vi "Datacluster remove duplicates_sort.vi"(6 "tolerance":dbl=0.0005 format="%.3e", 7 "ascending":bool, 9 "Sort?":bool, 10 "Datasets to be processed":T3(array[cluster])=[{"String"="KR6_Rh3In3Ge4", "Boolean"=TRUE, "begin"=0, "length"=99, "y weight"=1.0}], 11 "data cluster":cluster{"all rows":dbl[][]}[](array[cluster])=[{"all rows"=[[292.0, 292.9164, 75.02219, 292.5198, 292.873, 0.08675399, 165.5123, 4.898979, 292.4821, 292.7706, 292.492, 292.5008, 293.2383, 292.873, 25.04327, 12.87815, 8.722502e-06, 147301.0, 0.0, 49.12202, 7.026817e-06], [292.0, 292.6799, 51.88008, 291.997, 292.6172, 0.1254523, 164.8345, 4.898979, 291.9992, 292.2308, 292.069, 291.9987, 292.9044, 292.6172, 16.68079, 8.502932, 7.87955e-06, 148972.5, 0.0, 52.73522, 7.82408e-06], [289.0, 289.5872, 53.36827, 288.998, 289.5262, 0.121954, 164.6135, 4.898979, 288.9966, 289.0375, 288.9818, 288.9977, 289.7039, 289.5262, 16.9019, 8.586199, 8.115929e-06, 149524.0, 0.0, 53.28857, 7.979706e-06], [286.0, 286.5259, 49.68945, 285.998, 286.4604, 0.130983, 164.4479, 4.898979, 285.9991, 285.8497, 285.9015, 285.9993, 286.5396, 286.4604, 16.3069, 8.351839, 7.550718e-06, 150070.2, 0.0, 49.26372, 7.019865e-06], [283.0, 283.4711, 53.72872, 283.0, 283.4105, 0.1211359, 164.3414, 4.898979, 282.9993, 282.7069, 282.8492, 283.0001, 283.3894, 283.4105, 16.49914, 8.324846, 8.321034e-06, 150632.6, 0.0, 53.01569, 7.9647e-06], [280.0, 280.4225, 55.74425, 280.001, 280.3641, 0.116756, 164.0834, 4.898979, 279.9989, 279.5874, 279.805, 279.9995, 280.2632, 280.3641, 16.65599, 8.355238, 8.692565e-06, 151182.8, 0.0, 57.0127, 8.356655e-06], [277.0, 277.4087, 53.59749, 277.0, 277.348, 0.1214324, 163.8697, 4.898979, 276.999, 276.4814, 276.7861, 277.0003, 277.1648, 277.348, 16.48811, 8.322479, 8.417088e-06, 151713.2, 0.0, 56.02918, 8.50766e-06], [274.0, 274.42, 54.6898, 274.001, 274.3605, 0.1190071, 163.7107, 4.898979, 273.9996, 273.4294, 273.7956, 274.0001, 274.1133, 274.3605, 16.45529, 8.266658, 8.774592e-06, 152257.0, 0.0, 55.53214, 8.58475e-06], [271.0, 271.4452, 55.7095, 271.001, 271.3868, 0.1168288, 163.585, 4.898979, 270.9994, 270.3922, 270.812, 270.9999, 271.0838, 271.3868, 16.27431, 8.125881, 8.904832e-06, 152814.4, 0.0, 56.2198, 8.635062e-06], [268.0, 268.4699, 56.23065, 268.001, 268.412, 0.115746, 163.4811, 4.898979, 267.9992, 267.3543, 267.8305, 267.9997, 268.0515, 268.412, 16.14259, 8.031859, 9.125312e-06, 153358.0, 0.0, 56.47631, 9.315139e-06], [265.0, 265.504, 56.7819, 265.0, 265.4467, 0.1146223, 163.391, 4.898979, 264.9995, 264.3426, 264.8619, 264.9997, 265.042, 265.4467, 16.08378, 7.981424, 9.334535e-06, 153898.2, 0.0, 56.33507, 9.071532e-06], [262.0, 262.5402, 56.3029, 261.999, 262.4824, 0.1155975, 163.3034, 4.898979, 261.9999, 261.3382, 261.8933, 262.0, 262.0429, 262.4824, 15.96119, 7.921869, 9.410211e-06, 154447.6, 0.0, 56.37045, 9.069828e-06], [259.0, 259.5962, 58.10709, 259.0, 259.5401, 0.1120083, 163.2193, 4.898979, 258.9994, 258.3609, 258.9463, 258.9997, 259.0668, 259.5401, 15.93857, 7.860623, 9.705625e-06, 154984.0, 0.0, 56.57644, 9.146704e-06], [256.0, 256.6687, 56.23365, 255.999, 256.6109, 0.1157399, 163.1493, 4.898979, 255.999, 255.398, 256.0085, 255.9989, 256.1162, 256.6109, 15.6581, 7.744409, 9.492895e-06, 155529.5, 0.0, 56.48109, 9.279682e-06], [253.0, 253.5733, 56.38813, 253.0, 253.53, 0.08656709, 163.0587, 4.242641, 252.9989, 252.4462, 253.0724, 252.9998, 252.9904, 253.53, 15.52846, 7.664103, 9.532705e-06, 156076.4, 0.0, 55.89689, 9.252784e-06], [250.0, 250.6412, 54.69462, 250.0, 250.5966, 0.08924747, 162.9786, 4.242641, 250.0002, 249.4823, 250.1305, 250.0004, 250.0376, 250.5966, 15.19496, 7.512066, 9.061377e-06, 156639.2, 0.0, 56.67262, 9.431853e-06], [247.0, 247.7008, 56.19418, 247.001, 247.6573, 0.08686587, 162.8957, 4.242641, 246.9987, 246.5324, 247.1849, 247.0003, 247.0917, 247.6573, 15.12285, 7.431846, 9.658179e-06, 157187.5, 0.0, 58.88652, 9.951588e-06], [244.0, 244.756, 57.27194, 243.999, 244.7134, 0.08523119, 162.8167, 4.242641, 243.9985, 243.5809, 244.2381, 243.9991, 244.1415, 244.7134, 15.06449, 7.372421, 1.015879e-05, 157736.6, 0.0, 57.34745, 9.89733e-06], [241.0, 241.8457, 56.35606, 240.999, 241.8024, 0.08661635, 162.7319, 4.242641, 240.9999, 240.6596, 241.3181, 240.9994, 241.2305, 241.8024, 14.76138, 7.218644, 1.001309e-05, 158281.2, 0.0, 55.59713, 9.467991e-06], [238.0, 238.9209, 56.78944, 238.0, 238.8779, 0.08595534, 162.6528, 4.242641, 237.9983, 237.7335, 238.3869, 237.9997, 238.3104, 238.8779, 14.65413, 7.147241, 9.925203e-06, 158821.8, 0.0, 57.4055, 9.991189e-06], [235.0, 235.8546, 58.50336, 235.0, 235.8233, 0.0625779, 162.5361, 3.674235, 234.9997, 234.8069, 235.452, 234.9992, 235.2407, 235.8233, 14.56547, 7.060409, 1.032292e-05, 159362.6, 0.0, 58.88609, 1.077016e-05], [232.0, 232.9135, 58.7887, 232.0, 232.8823, 0.06227416, 162.4497, 3.674235, 231.9992, 231.8697, 232.505, 232.0, 232.3093, 232.8823, 14.4148, 6.969601, 1.039831e-05, 159894.4, 0.0, 60.38943, 1.099243e-05], [229.0, 229.9683, 52.90027, 228.999, 229.9337, 0.06920602, 162.3651, 3.674235, 228.9996, 228.9262, 229.5497, 228.9995, 229.3795, 229.9337, 13.95679, 6.834046, 9.47672e-06, 160443.8, 0.0, 55.18934, 1.011709e-05], [226.0, 227.0314, 55.01033, 226.001, 226.9982, 0.06655145, 162.2802, 3.674235, 225.9986, 225.9999, 226.6072, 226.0003, 226.4574, 226.9982, 13.87658, 6.741458, 1.003314e-05, 160986.4, 0.0, 56.71966, 9.916942e-06], [223.0, 224.0942, 54.51703, 222.999, 224.0606, 0.06715364, 162.193, 3.674235, 222.9989, 223.0755, 223.6635, 222.999, 223.5397, 224.0606, 13.63051, 6.611919, 9.828761e-06, 161551.5, 0.0, 57.5095, 1.147469e-05], [220.0, 221.1488, 53.22712, 219.999, 221.1144, 0.06878105, 162.1079, 3.674235, 219.9987, 220.1357, 220.7061, 219.9996, 220.6128, 221.1144, 13.28219, 6.44084, 9.954398e-06, 162102.9, 0.0, 56.94044, 1.050179e-05], [217.0, 218.18, 55.6197, 217.0, 218.1471, 0.06582231, 162.0181, 3.674235, 216.9999, 217.1911, 217.7388, 216.9998, 217.6652, 218.1471, 13.33998, 6.426719, 1.030691e-05, 162650.0, 0.0, 54.95497, 1.056938e-05], [214.0, 215.2041, 52.74785, 214.001, 215.1694, 0.069406, 161.9245, 3.674235, 213.9993, 214.2305, 214.7574, 214.0001, 214.7119, 215.1694, 13.16094, 6.381908, 1.041787e-05, 163183.7, 0.0, 54.82949, 1.00501e-05], [211.0, 212.2438, 53.2594, 210.999, 212.2094, 0.06873936, 161.8459, 3.674235, 211.0002, 211.2871, 211.7895, 210.9995, 211.7758, 212.2094, 12.92852, 6.240668, 1.038931e-05, 163737.5, 0.0, 53.69054, 9.725446e-06], [208.0, 209.2728, 54.18705, 208.0, 209.239, 0.06756258, 161.7569, 3.674235, 207.9997, 208.341, 208.8189, 207.9994, 208.8287, 209.239, 12.96622, 6.244319, 1.030433e-05, 164296.5, 0.0, 51.99244, 9.937355e-06], [205.0, 206.3015, 47.85468, 204.999, 206.2633, 0.0765028, 161.669, 3.674235, 204.9996, 205.3777, 205.8335, 204.9997, 205.8839, 206.2633, 12.49721, 6.108157, 8.850608e-06, 164832.5, 0.0, 52.33099, 1.025279e-05], [202.0, 203.3115, 47.77909, 202.0, 203.2732, 0.07662382, 161.578, 3.674235, 201.9992, 202.4024, 202.836, 201.9998, 202.9163, 203.2732, 12.32563, 6.011273, 9.175306e-06, 165383.8, 0.0, 49.48042, 9.796374e-06], [199.0, 200.3016, 48.81196, 199.001, 200.2641, 0.07500245, 161.4837, 3.674235, 198.9994, 199.4091, 199.8188, 199.0009, 199.9294, 200.2641, 12.19196, 5.913105, 9.19541e-06, 165931.2, 0.0, 48.99235, 9.119814e-06], [196.0, 197.3124, 46.33101, 196.0, 197.2728, 0.07901871, 161.3904, 3.674235, 195.9999, 196.4343, 196.8208, 195.9996, 196.9654, 197.2728, 11.90443, 5.801792, 9.14851e-06, 166481.8, 0.0, 47.56836, 9.084771e-06], [193.0, 194.3294, 48.48906, 193.0, 194.2917, 0.07550192, 161.2938, 3.674235, 192.9996, 193.4505, 193.8166, 192.9997, 194.001, 194.2917, 11.49295, 5.526408, 9.320439e-06, 167039.8, 0.0, 49.01581, 9.34799e-06], [190.0, 191.3157, 47.75745, 189.999, 191.2773, 0.07665855, 161.2094, 3.674235, 190.0005, 190.4523, 190.7964, 189.9991, 191.0099, 191.2773, 11.31843, 5.442408, 9.51165e-06, 167586.2, 0.0, 47.72681, 9.290438e-06], [187.0, 188.2909, 46.66995, 186.998, 188.2517, 0.07844485, 161.1183, 3.674235, 186.9996, 187.4401, 187.7654, 187.0006, 188.0048, 188.2517, 11.22194, 5.408542, 9.210011e-06, 168125.0, 0.0, 47.7442, 9.335471e-06], [184.0, 185.2608, 45.59003, 184.0, 185.2207, 0.08030301, 161.02, 3.674235, 183.9996, 184.4185, 184.7246, 183.9997, 184.9949, 185.2207, 10.97692, 5.291597, 8.987941e-06, 168671.0, 0.0, 45.18603, 8.882518e-06], [181.0, 182.2488, 42.55964, 181.0, 182.2057, 0.08602087, 160.9233, 3.674235, 180.9996, 181.4114, 181.7032, 180.9994, 182.0001, 182.2057, 10.7433, 5.21988, 8.481294e-06, 169224.8, 0.0, 42.92117, 8.932989e-06], [178.0, 179.2327, 43.4817, 178.0, 179.1906, 0.08419672, 160.8244, 3.674235, 177.9992, 178.3866, 178.6756, 177.9989, 178.9857, 179.1906, 10.55317, 5.093926, 8.674955e-06, 169761.4, 0.0, 46.08075, 9.801831e-06], [175.0, 176.1988, 41.91763, 174.999, 176.1551, 0.08733836, 160.7272, 3.674235, 174.9992, 175.3492, 175.6323, 175.0005, 175.9594, 176.1551, 10.39018, 5.032765, 8.418331e-06, 170337.0, 0.0, 41.27729, 8.256854e-06], [172.0, 173.1462, 40.78401, 171.998, 173.1014, 0.08976599, 160.6309, 3.674235, 171.9994, 172.2934, 172.5681, 172.0007, 172.9165, 173.1014, 10.17369, 4.933174, 8.561175e-06, 170884.7, 0.0, 42.0311, 8.954053e-06], [169.0, 170.1156, 39.52542, 169.002, 170.0692, 0.09262438, 160.5319, 3.674235, 168.9985, 169.2597, 169.5281, 169.0004, 169.8935, 170.0692, 10.01111, 4.866947, 7.889127e-06, 171427.6, 0.0, 41.17875, 8.476864e-06], [166.0, 167.0848, 37.75683, 166.0, 167.0363, 0.09696304, 160.4351, 3.674235, 165.9992, 166.2177, 166.4835, 165.9991, 166.8676, 167.0363, 9.732579, 4.745978, 7.667965e-06, 171976.2, 0.0, 40.17138, 7.923543e-06], [163.0, 164.0348, 37.48756, 163.0, 163.986, 0.09765951, 160.3364, 3.674235, 162.9994, 163.1585, 163.4224, 162.9994, 163.8198, 163.986, 9.565177, 4.656068, 7.403833e-06, 172519.0, 0.0, 37.92251, 7.706918e-06], [160.0, 160.9789, 37.24322, 160.0, 160.9297, 0.09830023, 160.2345, 3.674235, 159.9997, 160.0851, 160.3523, 159.9997, 160.7607, 160.9297, 9.362346, 4.545693, 7.846706e-06, 173077.8, 0.0, 38.13007, 8.027448e-06], [157.0, 157.7978, 36.56221, 157.0, 157.7603, 0.07509838, 160.1422, 3.181981, 157.0001, 157.0355, 157.3161, 157.0001, 157.5547, 157.7603, 9.136679, 4.431653, 7.299468e-06, 173622.6, 0.0, 36.74182, 7.431135e-06], [154.0, 154.7562, 36.11287, 153.999, 154.7182, 0.0760328, 160.039, 3.181981, 154.0002, 153.9788, 154.2641, 153.9991, 154.5089, 154.7182, 8.931389, 4.324545, 7.829839e-06, 174165.6, 0.0, 37.11626, 7.907207e-06], [151.0, 151.7025, 35.56308, 151.001, 151.6639, 0.07720823, 159.94, 3.181981, 150.9997, 150.9063, 151.1997, 151.0003, 151.4478, 151.6639, 8.772177, 4.245581, 7.074522e-06, 174712.4, 0.0, 34.8322, 7.606191e-06], [148.0, 148.6425, 34.07633, 148.001, 148.6022, 0.08057683, 159.8368, 3.181981, 148.0007, 147.8203, 148.1272, 148.0007, 148.376, 148.6022, 8.538666, 4.143502, 7.012669e-06, 175270.5, 0.0, 35.5259, 7.773223e-06], [145.0, 145.6151, 32.94494, 145.0, 145.5734, 0.08334398, 159.7329, 3.181981, 144.9995, 144.7711, 145.0917, 145.0, 145.3362, 145.5734, 8.402115, 4.089585, 6.717016e-06, 175825.6, 0.0, 34.5873, 7.462285e-06], [142.0, 142.4503, 32.69128, 141.998, 142.4188, 0.062993, 159.6235, 2.755676, 141.9999, 141.7087, 142.045, 141.998, 142.1454, 142.4188, 8.112161, 3.93007, 6.970786e-06, 176365.9, 0.0, 33.20516, 7.879391e-06], [139.0, 139.3994, 31.76623, 139.001, 139.367, 0.06482741, 159.5169, 2.755676, 138.9981, 138.6308, 138.9849, 138.9994, 139.0777, 139.367, 7.985541, 3.877216, 6.982463e-06, 176903.8, 0.0, 32.45839, 6.596733e-06], [136.0, 136.3652, 31.01851, 135.998, 136.332, 0.0663901, 159.4101, 2.755676, 135.9989, 135.5674, 135.9417, 135.999, 136.0241, 136.332, 7.79429, 3.784086, 6.795836e-06, 177452.3, 0.0, 32.19581, 6.462182e-06], [133.0, 133.3502, 30.5601, 133.0, 133.3165, 0.06738596, 159.3015, 2.755676, 132.9992, 132.5206, 132.9147, 132.9999, 132.9898, 133.3165, 7.59515, 3.680558, 6.903421e-06, 178000.4, 0.0, 31.58324, 6.744551e-06], [130.0, 130.2115, 29.16558, 130.0, 130.185, 0.05295598, 159.122, 2.386485, 130.0005, 129.4585, 129.875, 129.9997, 129.8214, 130.185, 7.33831, 3.563506, 7.084772e-06, 178528.9, 0.0, 30.31422, 6.637657e-06], [127.0, 127.0902, 28.66261, 127.0, 127.07, 0.04041393, 159.0379, 2.066757, 126.9998, 126.3926, 126.8334, 126.9993, 126.6696, 127.07, 7.211448, 3.501876, 6.550803e-06, 179072.6, 0.0, 27.84635, 6.955272e-06], [124.0, 124.092, 28.58992, 124.0, 124.0717, 0.04051669, 158.9287, 2.066757, 124.0006, 123.3645, 123.8279, 123.9994, 123.6488, 124.0717, 7.012868, 3.390962, 7.173261e-06, 179624.9, 0.0, 28.22442, 4.92486e-06], [121.0, 121.0173, 26.81918, 120.999, 121.0011, 0.03239384, 158.8124, 1.789864, 120.9991, 120.3247, 120.8123, 120.9995, 120.5459, 121.0011, 6.797255, 3.304885, 4.45575e-06, 180140.8, 0.0, 29.19013, 5.915953e-06], [118.0, 117.9932, 25.80576, 117.999, 117.9764, 0.03366599, 158.6989, 1.789864, 117.9995, 117.2703, 117.781, 118.0, 117.4994, 117.9764, 6.568201, 3.195852, 5.482144e-06, 180683.1, 0.0, 27.08986, 6.913137e-06], [115.0, 115.0141, 25.65538, 114.998, 114.9971, 0.03386332, 158.5865, 1.789864, 115.0005, 114.2643, 114.7982, 114.9996, 114.497, 114.9971, 6.423356, 3.116589, 5.528924e-06, 181217.8, 0.0, 26.62919, 5.253105e-06], [112.0, 112.0203, 26.59349, 112.001, 112.004, 0.03266877, 158.4708, 1.789864, 111.9995, 111.2424, 111.7992, 111.9994, 111.4798, 112.004, 6.320665, 3.040642, 5.840544e-06, 181744.4, 0.0, 26.32533, 6.485414e-06], [109.0, 109.016, 25.89338, 109.0, 108.9992, 0.03355207, 158.3582, 1.789864, 109.0002, 108.2095, 108.7884, 108.9998, 108.4539, 108.9992, 6.13315, 2.948822, 4.976681e-06, 182293.6, 0.0, 25.56833, 6.586255e-06], [106.0, 106.0601, 24.74948, 105.999, 106.0426, 0.03510282, 158.2417, 1.789864, 106.0009, 105.2233, 105.8221, 105.9986, 105.4789, 106.0426, 5.82098, 2.795607, 5.520496e-06, 182820.9, 0.0, 25.1926, 5.082759e-06], [103.0, 103.1012, 23.47957, 102.999, 103.0827, 0.03700138, 158.1265, 1.789864, 102.9994, 102.2249, 102.852, 102.9995, 102.4926, 103.0827, 5.610787, 2.701479, 5.748678e-06, 183358.4, 0.0, 24.56658, 4.990891e-06], [100.0, 100.1194, 24.40213, 100.0, 100.1016, 0.03560248, 158.0093, 1.789864, 99.99963, 99.21942, 99.86005, 99.99973, 99.49659, 100.1016, 5.418124, 2.579388, 5.193695e-06, 183898.6, 0.0, 24.73305, 4.828259e-06], [97.0, 97.17382, 23.39176, 97.0015, 97.15525, 0.03714027, 157.8955, 1.789864, 96.99884, 96.25454, 96.90598, 96.99946, 96.54095, 97.15525, 5.252876, 2.504921, 5.62191e-06, 184439.7, 0.0, 23.73066, 5.229691e-06], [94.0, 94.20774, 23.22087, 94.0002, 94.18903, 0.0374136, 157.7782, 1.789864, 93.99808, 93.27039, 93.92858, 94.00004, 93.56826, 94.18903, 5.073145, 2.409457, 5.538685e-06, 184984.4, 0.0, 23.61211, 6.687232e-06], [91.0, 91.13359, 22.59694, 91.0003, 91.11917, 0.02883498, 157.6522, 1.550068, 91.0004, 90.31659, 90.91559, 90.9996, 90.54901, 91.11917, 4.827745, 2.285596, 4.255465e-06, 185533.6, 0.0, 21.92768, 5.296259e-06], [88.0, 88.18123, 22.48137, 87.9991, 88.16674, 0.02898322, 157.5325, 1.550068, 87.9996, 87.35154, 87.95371, 87.99927, 87.59355, 88.16674, 4.645815, 2.189353, 4.903361e-06, 186084.2, 0.0, 21.34062, 6.20428e-06], [85.0, 85.24232, 22.00163, 84.9979, 85.22751, 0.02961518, 157.4127, 1.550068, 85.00029, 84.40605, 85.0051, 84.99872, 84.65807, 85.22751, 4.439868, 2.085645, 3.898806e-06, 186641.8, 0.0, 20.03455, 4.048067e-06], [82.0, 82.2906, 20.26436, 82.0003, 82.27452, 0.0321541, 157.2935, 1.550068, 81.99943, 81.3944, 82.04882, 81.99944, 81.65225, 82.27452, 4.366601, 2.069786, 4.384861e-06, 187170.4, 0.0, 19.93068, 5.169709e-06], [79.0, 79.35992, 20.65986, 78.9998, 79.34415, 0.03153857, 157.175, 1.550068, 78.99976, 78.46501, 79.10271, 78.99972, 78.73799, 79.34415, 4.123809, 1.934396, 5.660535e-06, 187707.0, 0.0, 20.24228, 3.521332e-06], [76.0, 76.34799, 18.14755, 76.0001, 76.33453, 0.02692852, 157.0442, 1.342398, 75.9988, 75.52364, 76.14176, 76.00082, 75.74333, 76.33453, 3.879228, 1.836679, 5.277406e-06, 188227.8, 0.0, 18.3202, 4.280038e-06], [73.0, 73.40674, 18.83722, 72.9989, 73.39377, 0.02594261, 156.9286, 1.342398, 72.9991, 72.60294, 73.19315, 72.99918, 72.82951, 73.39377, 3.728216, 1.746902, 4.133453e-06, 188764.6, 0.0, 20.32012, 4.874801e-06], [70.0, 70.45695, 17.51673, 70.0003, 70.443, 0.02789829, 156.8115, 1.342398, 70.00086, 69.67221, 70.23128, 69.99956, 69.91183, 70.443, 3.505012, 1.644658, 3.415282e-06, 189312.8, 0.0, 18.10538, 3.636672e-06], [67.0, 67.51137, 17.06142, 66.9986, 67.49705, 0.0286428, 156.6926, 1.342398, 67.0003, 66.75251, 67.27265, 66.99976, 67.00556, 67.49705, 3.329935, 1.557489, 3.637388e-06, 189850.0, 0.0, 17.81273, 2.997229e-06], [64.0, 64.55299, 16.05667, 63.9994, 64.53777, 0.03043512, 156.572, 1.342398, 63.99965, 63.82388, 64.3001, 64.00019, 64.09199, 64.53777, 3.155975, 1.477454, 3.836114e-06, 190372.4, 0.0, 16.65761, 3.137167e-06], [61.0, 61.59684, 15.15327, 61.0012, 61.58071, 0.03224959, 156.4552, 1.342398, 61.00003, 60.89696, 61.32582, 60.99921, 61.18411, 61.58071, 2.932403, 1.370073, 2.715446e-06, 190890.4, 0.0, 15.46223, 4.794554e-06], [58.0, 58.6279, 14.0184, 58.0008, 58.61047, 0.03486038, 156.3434, 1.342398, 57.99915, 57.96364, 58.33762, 57.99934, 58.27135, 58.61047, 2.745862, 1.284894, 2.94282e-06, 191408.4, 0.0, 14.4151, 4.772166e-06], [55.0, 55.65962, 12.33515, 55.0029, 55.63981, 0.03961743, 156.2312, 1.342398, 54.99762, 55.02696, 55.34105, 55.0008, 55.36534, 55.63981, 2.519189, 1.185287, 3.164869e-06, 191919.5, 0.0, 12.86659, 1.828514e-06], [52.0, 52.69421, 11.21244, 51.999, 52.67242, 0.04358434, 156.12, 1.342398, 51.99888, 52.0955, 52.34609, 51.99949, 52.46542, 52.67242, 2.286444, 1.075562, 2.081657e-06, 192439.7, 0.0, 11.76603, 2.789106e-06], [49.0, 49.61418, 9.645293, 49.001, 49.59518, 0.03799937, 156.0042, 1.162551, 48.99919, 49.13845, 49.32293, 49.00038, 49.4487, 49.59518, 2.049105, 0.9693383, 2.419945e-06, 192925.6, 0.0, 10.21014, 2.551699e-06], [46.0, 46.64398, 8.849838, 46.0014, 46.62327, 0.04141489, 155.8991, 1.162551, 45.99971, 46.20159, 46.31906, 45.99925, 46.54721, 46.62327, 1.829977, 0.8624549, 2.062263e-06, 193484.8, 0.0, 8.642792, 8.766135e-07], [43.0, 43.63805, 8.111564, 43.0, 43.61546, 0.04518427, 155.7963, 1.162551, 43.00087, 43.23263, 43.28277, 42.99939, 43.6105, 43.61546, 1.669476, 0.7863123, 2.202847e-06, 194031.9, 0.0, 8.304894, 2.187056e-06], [40.0, 40.60721, 7.850611, 39.9976, 40.58387, 0.04668618, 155.6928, 1.162551, 39.99903, 40.24392, 40.22946, 39.99922, 40.64502, 40.58387, 1.579687, 0.7417823, 1.934699e-06, 194511.3, 0.0, 7.823251, 1.052641e-06], [37.0, 37.55588, 7.570818, 37.0021, 37.53168, 0.04841156, 155.5887, 1.162551, 36.99997, 37.23081, 37.15568, 36.99985, 37.65521, 37.53168, 1.491856, 0.6986331, 1.616464e-06, 195029.6, 0.0, 7.701154, 1.426829e-06], [34.0, 34.39013, 7.129456, 34.002, 34.37085, 0.03855642, 155.4653, 1.006799, 34.00288, 34.19961, 34.07078, 33.99971, 34.53824, 34.37085, 1.389701, 0.6498903, 1.456064e-06, 195501.9, 0.0, 7.197325, 1.830936e-06], [31.0, 31.3295, 6.959681, 30.9971, 31.30975, 0.03949697, 155.3693, 1.006799, 31.00027, 31.15947, 30.98673, 30.99905, 31.52198, 31.30975, 1.305866, 0.6077944, 1.746532e-06, 195974.6, 0.0, 6.855044, 1.3535e-07], [28.0, 28.257, 6.444445, 28.0083, 28.23568, 0.04265477, 155.2754, 1.006799, 27.99751, 28.08427, 27.88122, 28.00025, 28.48138, 28.23568, 1.20443, 0.5603139, 1.207888e-06, 196438.7, 0.0, 6.465166, 2.29124e-06], [25.0, 25.1858, 5.908139, 25.0055, 25.16253, 0.04652672, 155.1906, 1.006799, 25.00147, 24.99086, 24.77406, 24.99832, 25.42586, 25.16253, 1.084087, 0.5032175, 9.614257e-07, 196931.6, 0.0, 5.92471, -5.51895e-08], [22.0, 22.16916, 5.305623, 21.9854, 22.14325, 0.05181037, 155.1142, 1.006799, 22.00671, 21.91764, 21.70696, 21.99982, 22.40575, 22.14325, 0.959603, 0.4446781, 7.916026e-07, 197380.4, 0.0, 5.277611, 2.768679e-07], [19.0, 19.30572, 4.637635, 18.9844, 19.27608, 0.05927295, 155.0499, 1.006799, 18.99661, 18.95241, 18.76765, 19.00061, 19.52011, 19.27608, 0.8426237, 0.390679, 5.587576e-07, 197860.4, 0.0, 4.670142, -7.621961e-08], [16.0, 16.50024, 3.972702, 16.0034, 16.46565, 0.06919378, 154.9962, 1.006799, 15.99681, 16.00464, 15.86607, 15.99389, 16.67341, 16.46565, 0.7071578, 0.3270905, 3.955843e-07, 198345.2, 0.0, 3.981336, -9.093087e-09], [13.0, 13.71888, 3.255681, 13.0265, 13.67666, 0.08443282, 154.9529, 1.006799, 12.99021, 12.98951, 12.9155, 12.99523, 13.83511, 13.67666, 0.5650661, 0.2606204, 4.899574e-08, 199058.5, 0.0, 3.267024, -3.089664e-07], [10.0, 11.02144, 2.634719, 9.9178, 10.96927, 0.1043323, 154.9244, 1.006799, 9.979209, 9.944225, 9.937939, 9.981572, 11.07989, 10.96927, 0.4191188, 0.1915213, 3.509129e-08, 199788.6, 0.0, 2.637912, 3.892924e-07], [7.0, 8.207977, 2.280254, 7.0263, 8.162771, 0.09041306, 154.877, 0.8719131, 6.996675, 6.899136, 6.944581, 6.995916, 8.207738, 8.162771, 0.272072, 0.1212537, 1.590448e-07, 200474.8, 0.0, 2.226699, -2.06841e-07], [4.0, 6.17061, 6.914511, 3.9852, 6.155702, 0.02981624, 154.8519, 0.8719131, 4.007358, 3.946248, 3.912001, 4.007225, 6.219766, 6.155702, 0.1566822, 0.06587024, 3.496313e-07, 201190.7, 0.0, 6.388795, -3.268214e-08], [2.0, 3.439481, -0.8426919, 2.2818, 3.470062, -0.06116255, 154.8119, 0.4359565, 2.275721, 2.314741, 2.136495, 2.275818, 3.587147, 3.470062, 0.06999886, 0.02771, -3.623877e-09, 201712.2, 0.0, -0.8426919, -3.623877e-09]]}]) -> (3 "data cluster out":cluster{"all rows":dbl[][]}[](array[cluster])=[{"all rows"=[[292.0, 292.9164, 75.02219, 292.5198, 292.873, 0.08675399, 165.5123, 4.898979, 292.4821, 292.7706, 292.492, 292.5008, 293.2383, 292.873, 25.04327, 12.87815, 8.722502e-06, 147301.0, 0.0, 49.12202, 7.026817e-06], [292.0, 292.6799, 51.88008, 291.997, 292.6172, 0.1254523, 164.8345, 4.898979, 291.9992, 292.2308, 292.069, 291.9987, 292.9044, 292.6172, 16.68079, 8.502932, 7.87955e-06, 148972.5, 0.0, 52.73522, 7.82408e-06], [289.0, 289.5872, 53.36827, 288.998, 289.5262, 0.121954, 164.6135, 4.898979, 288.9966, 289.0375, 288.9818, 288.9977, 289.7039, 289.5262, 16.9019, 8.586199, 8.115929e-06, 149524.0, 0.0, 53.28857, 7.979706e-06], [286.0, 286.5259, 49.68945, 285.998, 286.4604, 0.130983, 164.4479, 4.898979, 285.9991, 285.8497, 285.9015, 285.9993, 286.5396, 286.4604, 16.3069, 8.351839, 7.550718e-06, 150070.2, 0.0, 49.26372, 7.019865e-06], [283.0, 283.4711, 53.72872, 283.0, 283.4105, 0.1211359, 164.3414, 4.898979, 282.9993, 282.7069, 282.8492, 283.0001, 283.3894, 283.4105, 16.49914, 8.324846, 8.321034e-06, 150632.6, 0.0, 53.01569, 7.9647e-06], [280.0, 280.4225, 55.74425, 280.001, 280.3641, 0.116756, 164.0834, 4.898979, 279.9989, 279.5874, 279.805, 279.9995, 280.2632, 280.3641, 16.65599, 8.355238, 8.692565e-06, 151182.8, 0.0, 57.0127, 8.356655e-06], [277.0, 277.4087, 53.59749, 277.0, 277.348, 0.1214324, 163.8697, 4.898979, 276.999, 276.4814, 276.7861, 277.0003, 277.1648, 277.348, 16.48811, 8.322479, 8.417088e-06, 151713.2, 0.0, 56.02918, 8.50766e-06], [274.0, 274.42, 54.6898, 274.001, 274.3605, 0.1190071, 163.7107, 4.898979, 273.9996, 273.4294, 273.7956, 274.0001, 274.1133, 274.3605, 16.45529, 8.266658, 8.774592e-06, 152257.0, 0.0, 55.53214, 8.58475e-06], [271.0, 271.4452, 55.7095, 271.001, 271.3868, 0.1168288, 163.585, 4.898979, 270.9994, 270.3922, 270.812, 270.9999, 271.0838, 271.3868, 16.27431, 8.125881, 8.904832e-06, 152814.4, 0.0, 56.2198, 8.635062e-06], [268.0, 268.4699, 56.23065, 268.001, 268.412, 0.115746, 163.4811, 4.898979, 267.9992, 267.3543, 267.8305, 267.9997, 268.0515, 268.412, 16.14259, 8.031859, 9.125312e-06, 153358.0, 0.0, 56.47631, 9.315139e-06], [265.0, 265.504, 56.7819, 265.0, 265.4467, 0.1146223, 163.391, 4.898979, 264.9995, 264.3426, 264.8619, 264.9997, 265.042, 265.4467, 16.08378, 7.981424, 9.334535e-06, 153898.2, 0.0, 56.33507, 9.071532e-06], [262.0, 262.5402, 56.3029, 261.999, 262.4824, 0.1155975, 163.3034, 4.898979, 261.9999, 261.3382, 261.8933, 262.0, 262.0429, 262.4824, 15.96119, 7.921869, 9.410211e-06, 154447.6, 0.0, 56.37045, 9.069828e-06], [259.0, 259.5962, 58.10709, 259.0, 259.5401, 0.1120083, 163.2193, 4.898979, 258.9994, 258.3609, 258.9463, 258.9997, 259.0668, 259.5401, 15.93857, 7.860623, 9.705625e-06, 154984.0, 0.0, 56.57644, 9.146704e-06], [256.0, 256.6687, 56.23365, 255.999, 256.6109, 0.1157399, 163.1493, 4.898979, 255.999, 255.398, 256.0085, 255.9989, 256.1162, 256.6109, 15.6581, 7.744409, 9.492895e-06, 155529.5, 0.0, 56.48109, 9.279682e-06], [253.0, 253.5733, 56.38813, 253.0, 253.53, 0.08656709, 163.0587, 4.242641, 252.9989, 252.4462, 253.0724, 252.9998, 252.9904, 253.53, 15.52846, 7.664103, 9.532705e-06, 156076.4, 0.0, 55.89689, 9.252784e-06], [250.0, 250.6412, 54.69462, 250.0, 250.5966, 0.08924747, 162.9786, 4.242641, 250.0002, 249.4823, 250.1305, 250.0004, 250.0376, 250.5966, 15.19496, 7.512066, 9.061377e-06, 156639.2, 0.0, 56.67262, 9.431853e-06], [247.0, 247.7008, 56.19418, 247.001, 247.6573, 0.08686587, 162.8957, 4.242641, 246.9987, 246.5324, 247.1849, 247.0003, 247.0917, 247.6573, 15.12285, 7.431846, 9.658179e-06, 157187.5, 0.0, 58.88652, 9.951588e-06], [244.0, 244.756, 57.27194, 243.999, 244.7134, 0.08523119, 162.8167, 4.242641, 243.9985, 243.5809, 244.2381, 243.9991, 244.1415, 244.7134, 15.06449, 7.372421, 1.015879e-05, 157736.6, 0.0, 57.34745, 9.89733e-06], [241.0, 241.8457, 56.35606, 240.999, 241.8024, 0.08661635, 162.7319, 4.242641, 240.9999, 240.6596, 241.3181, 240.9994, 241.2305, 241.8024, 14.76138, 7.218644, 1.001309e-05, 158281.2, 0.0, 55.59713, 9.467991e-06], [238.0, 238.9209, 56.78944, 238.0, 238.8779, 0.08595534, 162.6528, 4.242641, 237.9983, 237.7335, 238.3869, 237.9997, 238.3104, 238.8779, 14.65413, 7.147241, 9.925203e-06, 158821.8, 0.0, 57.4055, 9.991189e-06], [235.0, 235.8546, 58.50336, 235.0, 235.8233, 0.0625779, 162.5361, 3.674235, 234.9997, 234.8069, 235.452, 234.9992, 235.2407, 235.8233, 14.56547, 7.060409, 1.032292e-05, 159362.6, 0.0, 58.88609, 1.077016e-05], [232.0, 232.9135, 58.7887, 232.0, 232.8823, 0.06227416, 162.4497, 3.674235, 231.9992, 231.8697, 232.505, 232.0, 232.3093, 232.8823, 14.4148, 6.969601, 1.039831e-05, 159894.4, 0.0, 60.38943, 1.099243e-05], [229.0, 229.9683, 52.90027, 228.999, 229.9337, 0.06920602, 162.3651, 3.674235, 228.9996, 228.9262, 229.5497, 228.9995, 229.3795, 229.9337, 13.95679, 6.834046, 9.47672e-06, 160443.8, 0.0, 55.18934, 1.011709e-05], [226.0, 227.0314, 55.01033, 226.001, 226.9982, 0.06655145, 162.2802, 3.674235, 225.9986, 225.9999, 226.6072, 226.0003, 226.4574, 226.9982, 13.87658, 6.741458, 1.003314e-05, 160986.4, 0.0, 56.71966, 9.916942e-06], [223.0, 224.0942, 54.51703, 222.999, 224.0606, 0.06715364, 162.193, 3.674235, 222.9989, 223.0755, 223.6635, 222.999, 223.5397, 224.0606, 13.63051, 6.611919, 9.828761e-06, 161551.5, 0.0, 57.5095, 1.147469e-05], [220.0, 221.1488, 53.22712, 219.999, 221.1144, 0.06878105, 162.1079, 3.674235, 219.9987, 220.1357, 220.7061, 219.9996, 220.6128, 221.1144, 13.28219, 6.44084, 9.954398e-06, 162102.9, 0.0, 56.94044, 1.050179e-05], [217.0, 218.18, 55.6197, 217.0, 218.1471, 0.06582231, 162.0181, 3.674235, 216.9999, 217.1911, 217.7388, 216.9998, 217.6652, 218.1471, 13.33998, 6.426719, 1.030691e-05, 162650.0, 0.0, 54.95497, 1.056938e-05], [214.0, 215.2041, 52.74785, 214.001, 215.1694, 0.069406, 161.9245, 3.674235, 213.9993, 214.2305, 214.7574, 214.0001, 214.7119, 215.1694, 13.16094, 6.381908, 1.041787e-05, 163183.7, 0.0, 54.82949, 1.00501e-05], [211.0, 212.2438, 53.2594, 210.999, 212.2094, 0.06873936, 161.8459, 3.674235, 211.0002, 211.2871, 211.7895, 210.9995, 211.7758, 212.2094, 12.92852, 6.240668, 1.038931e-05, 163737.5, 0.0, 53.69054, 9.725446e-06], [208.0, 209.2728, 54.18705, 208.0, 209.239, 0.06756258, 161.7569, 3.674235, 207.9997, 208.341, 208.8189, 207.9994, 208.8287, 209.239, 12.96622, 6.244319, 1.030433e-05, 164296.5, 0.0, 51.99244, 9.937355e-06], [205.0, 206.3015, 47.85468, 204.999, 206.2633, 0.0765028, 161.669, 3.674235, 204.9996, 205.3777, 205.8335, 204.9997, 205.8839, 206.2633, 12.49721, 6.108157, 8.850608e-06, 164832.5, 0.0, 52.33099, 1.025279e-05], [202.0, 203.3115, 47.77909, 202.0, 203.2732, 0.07662382, 161.578, 3.674235, 201.9992, 202.4024, 202.836, 201.9998, 202.9163, 203.2732, 12.32563, 6.011273, 9.175306e-06, 165383.8, 0.0, 49.48042, 9.796374e-06], [199.0, 200.3016, 48.81196, 199.001, 200.2641, 0.07500245, 161.4837, 3.674235, 198.9994, 199.4091, 199.8188, 199.0009, 199.9294, 200.2641, 12.19196, 5.913105, 9.19541e-06, 165931.2, 0.0, 48.99235, 9.119814e-06], [196.0, 197.3124, 46.33101, 196.0, 197.2728, 0.07901871, 161.3904, 3.674235, 195.9999, 196.4343, 196.8208, 195.9996, 196.9654, 197.2728, 11.90443, 5.801792, 9.14851e-06, 166481.8, 0.0, 47.56836, 9.084771e-06], [193.0, 194.3294, 48.48906, 193.0, 194.2917, 0.07550192, 161.2938, 3.674235, 192.9996, 193.4505, 193.8166, 192.9997, 194.001, 194.2917, 11.49295, 5.526408, 9.320439e-06, 167039.8, 0.0, 49.01581, 9.34799e-06], [190.0, 191.3157, 47.75745, 189.999, 191.2773, 0.07665855, 161.2094, 3.674235, 190.0005, 190.4523, 190.7964, 189.9991, 191.0099, 191.2773, 11.31843, 5.442408, 9.51165e-06, 167586.2, 0.0, 47.72681, 9.290438e-06], [187.0, 188.2909, 46.66995, 186.998, 188.2517, 0.07844485, 161.1183, 3.674235, 186.9996, 187.4401, 187.7654, 187.0006, 188.0048, 188.2517, 11.22194, 5.408542, 9.210011e-06, 168125.0, 0.0, 47.7442, 9.335471e-06], [184.0, 185.2608, 45.59003, 184.0, 185.2207, 0.08030301, 161.02, 3.674235, 183.9996, 184.4185, 184.7246, 183.9997, 184.9949, 185.2207, 10.97692, 5.291597, 8.987941e-06, 168671.0, 0.0, 45.18603, 8.882518e-06], [181.0, 182.2488, 42.55964, 181.0, 182.2057, 0.08602087, 160.9233, 3.674235, 180.9996, 181.4114, 181.7032, 180.9994, 182.0001, 182.2057, 10.7433, 5.21988, 8.481294e-06, 169224.8, 0.0, 42.92117, 8.932989e-06], [178.0, 179.2327, 43.4817, 178.0, 179.1906, 0.08419672, 160.8244, 3.674235, 177.9992, 178.3866, 178.6756, 177.9989, 178.9857, 179.1906, 10.55317, 5.093926, 8.674955e-06, 169761.4, 0.0, 46.08075, 9.801831e-06], [175.0, 176.1988, 41.91763, 174.999, 176.1551, 0.08733836, 160.7272, 3.674235, 174.9992, 175.3492, 175.6323, 175.0005, 175.9594, 176.1551, 10.39018, 5.032765, 8.418331e-06, 170337.0, 0.0, 41.27729, 8.256854e-06], [172.0, 173.1462, 40.78401, 171.998, 173.1014, 0.08976599, 160.6309, 3.674235, 171.9994, 172.2934, 172.5681, 172.0007, 172.9165, 173.1014, 10.17369, 4.933174, 8.561175e-06, 170884.7, 0.0, 42.0311, 8.954053e-06], [169.0, 170.1156, 39.52542, 169.002, 170.0692, 0.09262438, 160.5319, 3.674235, 168.9985, 169.2597, 169.5281, 169.0004, 169.8935, 170.0692, 10.01111, 4.866947, 7.889127e-06, 171427.6, 0.0, 41.17875, 8.476864e-06], [166.0, 167.0848, 37.75683, 166.0, 167.0363, 0.09696304, 160.4351, 3.674235, 165.9992, 166.2177, 166.4835, 165.9991, 166.8676, 167.0363, 9.732579, 4.745978, 7.667965e-06, 171976.2, 0.0, 40.17138, 7.923543e-06], [163.0, 164.0348, 37.48756, 163.0, 163.986, 0.09765951, 160.3364, 3.674235, 162.9994, 163.1585, 163.4224, 162.9994, 163.8198, 163.986, 9.565177, 4.656068, 7.403833e-06, 172519.0, 0.0, 37.92251, 7.706918e-06], [160.0, 160.9789, 37.24322, 160.0, 160.9297, 0.09830023, 160.2345, 3.674235, 159.9997, 160.0851, 160.3523, 159.9997, 160.7607, 160.9297, 9.362346, 4.545693, 7.846706e-06, 173077.8, 0.0, 38.13007, 8.027448e-06], [157.0, 157.7978, 36.56221, 157.0, 157.7603, 0.07509838, 160.1422, 3.181981, 157.0001, 157.0355, 157.3161, 157.0001, 157.5547, 157.7603, 9.136679, 4.431653, 7.299468e-06, 173622.6, 0.0, 36.74182, 7.431135e-06], [154.0, 154.7562, 36.11287, 153.999, 154.7182, 0.0760328, 160.039, 3.181981, 154.0002, 153.9788, 154.2641, 153.9991, 154.5089, 154.7182, 8.931389, 4.324545, 7.829839e-06, 174165.6, 0.0, 37.11626, 7.907207e-06], [151.0, 151.7025, 35.56308, 151.001, 151.6639, 0.07720823, 159.94, 3.181981, 150.9997, 150.9063, 151.1997, 151.0003, 151.4478, 151.6639, 8.772177, 4.245581, 7.074522e-06, 174712.4, 0.0, 34.8322, 7.606191e-06], [148.0, 148.6425, 34.07633, 148.001, 148.6022, 0.08057683, 159.8368, 3.181981, 148.0007, 147.8203, 148.1272, 148.0007, 148.376, 148.6022, 8.538666, 4.143502, 7.012669e-06, 175270.5, 0.0, 35.5259, 7.773223e-06], [145.0, 145.6151, 32.94494, 145.0, 145.5734, 0.08334398, 159.7329, 3.181981, 144.9995, 144.7711, 145.0917, 145.0, 145.3362, 145.5734, 8.402115, 4.089585, 6.717016e-06, 175825.6, 0.0, 34.5873, 7.462285e-06], [142.0, 142.4503, 32.69128, 141.998, 142.4188, 0.062993, 159.6235, 2.755676, 141.9999, 141.7087, 142.045, 141.998, 142.1454, 142.4188, 8.112161, 3.93007, 6.970786e-06, 176365.9, 0.0, 33.20516, 7.879391e-06], [139.0, 139.3994, 31.76623, 139.001, 139.367, 0.06482741, 159.5169, 2.755676, 138.9981, 138.6308, 138.9849, 138.9994, 139.0777, 139.367, 7.985541, 3.877216, 6.982463e-06, 176903.8, 0.0, 32.45839, 6.596733e-06], [136.0, 136.3652, 31.01851, 135.998, 136.332, 0.0663901, 159.4101, 2.755676, 135.9989, 135.5674, 135.9417, 135.999, 136.0241, 136.332, 7.79429, 3.784086, 6.795836e-06, 177452.3, 0.0, 32.19581, 6.462182e-06], [133.0, 133.3502, 30.5601, 133.0, 133.3165, 0.06738596, 159.3015, 2.755676, 132.9992, 132.5206, 132.9147, 132.9999, 132.9898, 133.3165, 7.59515, 3.680558, 6.903421e-06, 178000.4, 0.0, 31.58324, 6.744551e-06], [130.0, 130.2115, 29.16558, 130.0, 130.185, 0.05295598, 159.122, 2.386485, 130.0005, 129.4585, 129.875, 129.9997, 129.8214, 130.185, 7.33831, 3.563506, 7.084772e-06, 178528.9, 0.0, 30.31422, 6.637657e-06], [127.0, 127.0902, 28.66261, 127.0, 127.07, 0.04041393, 159.0379, 2.066757, 126.9998, 126.3926, 126.8334, 126.9993, 126.6696, 127.07, 7.211448, 3.501876, 6.550803e-06, 179072.6, 0.0, 27.84635, 6.955272e-06], [124.0, 124.092, 28.58992, 124.0, 124.0717, 0.04051669, 158.9287, 2.066757, 124.0006, 123.3645, 123.8279, 123.9994, 123.6488, 124.0717, 7.012868, 3.390962, 7.173261e-06, 179624.9, 0.0, 28.22442, 4.92486e-06], [121.0, 121.0173, 26.81918, 120.999, 121.0011, 0.03239384, 158.8124, 1.789864, 120.9991, 120.3247, 120.8123, 120.9995, 120.5459, 121.0011, 6.797255, 3.304885, 4.45575e-06, 180140.8, 0.0, 29.19013, 5.915953e-06], [118.0, 117.9932, 25.80576, 117.999, 117.9764, 0.03366599, 158.6989, 1.789864, 117.9995, 117.2703, 117.781, 118.0, 117.4994, 117.9764, 6.568201, 3.195852, 5.482144e-06, 180683.1, 0.0, 27.08986, 6.913137e-06], [115.0, 115.0141, 25.65538, 114.998, 114.9971, 0.03386332, 158.5865, 1.789864, 115.0005, 114.2643, 114.7982, 114.9996, 114.497, 114.9971, 6.423356, 3.116589, 5.528924e-06, 181217.8, 0.0, 26.62919, 5.253105e-06], [112.0, 112.0203, 26.59349, 112.001, 112.004, 0.03266877, 158.4708, 1.789864, 111.9995, 111.2424, 111.7992, 111.9994, 111.4798, 112.004, 6.320665, 3.040642, 5.840544e-06, 181744.4, 0.0, 26.32533, 6.485414e-06], [109.0, 109.016, 25.89338, 109.0, 108.9992, 0.03355207, 158.3582, 1.789864, 109.0002, 108.2095, 108.7884, 108.9998, 108.4539, 108.9992, 6.13315, 2.948822, 4.976681e-06, 182293.6, 0.0, 25.56833, 6.586255e-06], [106.0, 106.0601, 24.74948, 105.999, 106.0426, 0.03510282, 158.2417, 1.789864, 106.0009, 105.2233, 105.8221, 105.9986, 105.4789, 106.0426, 5.82098, 2.795607, 5.520496e-06, 182820.9, 0.0, 25.1926, 5.082759e-06], [103.0, 103.1012, 23.47957, 102.999, 103.0827, 0.03700138, 158.1265, 1.789864, 102.9994, 102.2249, 102.852, 102.9995, 102.4926, 103.0827, 5.610787, 2.701479, 5.748678e-06, 183358.4, 0.0, 24.56658, 4.990891e-06], [100.0, 100.1194, 24.40213, 100.0, 100.1016, 0.03560248, 158.0093, 1.789864, 99.99963, 99.21942, 99.86005, 99.99973, 99.49659, 100.1016, 5.418124, 2.579388, 5.193695e-06, 183898.6, 0.0, 24.73305, 4.828259e-06], [97.0, 97.17382, 23.39176, 97.0015, 97.15525, 0.03714027, 157.8955, 1.789864, 96.99884, 96.25454, 96.90598, 96.99946, 96.54095, 97.15525, 5.252876, 2.504921, 5.62191e-06, 184439.7, 0.0, 23.73066, 5.229691e-06], [94.0, 94.20774, 23.22087, 94.0002, 94.18903, 0.0374136, 157.7782, 1.789864, 93.99808, 93.27039, 93.92858, 94.00004, 93.56826, 94.18903, 5.073145, 2.409457, 5.538685e-06, 184984.4, 0.0, 23.61211, 6.687232e-06], [91.0, 91.13359, 22.59694, 91.0003, 91.11917, 0.02883498, 157.6522, 1.550068, 91.0004, 90.31659, 90.91559, 90.9996, 90.54901, 91.11917, 4.827745, 2.285596, 4.255465e-06, 185533.6, 0.0, 21.92768, 5.296259e-06], [88.0, 88.18123, 22.48137, 87.9991, 88.16674, 0.02898322, 157.5325, 1.550068, 87.9996, 87.35154, 87.95371, 87.99927, 87.59355, 88.16674, 4.645815, 2.189353, 4.903361e-06, 186084.2, 0.0, 21.34062, 6.20428e-06], [85.0, 85.24232, 22.00163, 84.9979, 85.22751, 0.02961518, 157.4127, 1.550068, 85.00029, 84.40605, 85.0051, 84.99872, 84.65807, 85.22751, 4.439868, 2.085645, 3.898806e-06, 186641.8, 0.0, 20.03455, 4.048067e-06], [82.0, 82.2906, 20.26436, 82.0003, 82.27452, 0.0321541, 157.2935, 1.550068, 81.99943, 81.3944, 82.04882, 81.99944, 81.65225, 82.27452, 4.366601, 2.069786, 4.384861e-06, 187170.4, 0.0, 19.93068, 5.169709e-06], [79.0, 79.35992, 20.65986, 78.9998, 79.34415, 0.03153857, 157.175, 1.550068, 78.99976, 78.46501, 79.10271, 78.99972, 78.73799, 79.34415, 4.123809, 1.934396, 5.660535e-06, 187707.0, 0.0, 20.24228, 3.521332e-06], [76.0, 76.34799, 18.14755, 76.0001, 76.33453, 0.02692852, 157.0442, 1.342398, 75.9988, 75.52364, 76.14176, 76.00082, 75.74333, 76.33453, 3.879228, 1.836679, 5.277406e-06, 188227.8, 0.0, 18.3202, 4.280038e-06], [73.0, 73.40674, 18.83722, 72.9989, 73.39377, 0.02594261, 156.9286, 1.342398, 72.9991, 72.60294, 73.19315, 72.99918, 72.82951, 73.39377, 3.728216, 1.746902, 4.133453e-06, 188764.6, 0.0, 20.32012, 4.874801e-06], [70.0, 70.45695, 17.51673, 70.0003, 70.443, 0.02789829, 156.8115, 1.342398, 70.00086, 69.67221, 70.23128, 69.99956, 69.91183, 70.443, 3.505012, 1.644658, 3.415282e-06, 189312.8, 0.0, 18.10538, 3.636672e-06], [67.0, 67.51137, 17.06142, 66.9986, 67.49705, 0.0286428, 156.6926, 1.342398, 67.0003, 66.75251, 67.27265, 66.99976, 67.00556, 67.49705, 3.329935, 1.557489, 3.637388e-06, 189850.0, 0.0, 17.81273, 2.997229e-06], [64.0, 64.55299, 16.05667, 63.9994, 64.53777, 0.03043512, 156.572, 1.342398, 63.99965, 63.82388, 64.3001, 64.00019, 64.09199, 64.53777, 3.155975, 1.477454, 3.836114e-06, 190372.4, 0.0, 16.65761, 3.137167e-06], [61.0, 61.59684, 15.15327, 61.0012, 61.58071, 0.03224959, 156.4552, 1.342398, 61.00003, 60.89696, 61.32582, 60.99921, 61.18411, 61.58071, 2.932403, 1.370073, 2.715446e-06, 190890.4, 0.0, 15.46223, 4.794554e-06], [58.0, 58.6279, 14.0184, 58.0008, 58.61047, 0.03486038, 156.3434, 1.342398, 57.99915, 57.96364, 58.33762, 57.99934, 58.27135, 58.61047, 2.745862, 1.284894, 2.94282e-06, 191408.4, 0.0, 14.4151, 4.772166e-06], [55.0, 55.65962, 12.33515, 55.0029, 55.63981, 0.03961743, 156.2312, 1.342398, 54.99762, 55.02696, 55.34105, 55.0008, 55.36534, 55.63981, 2.519189, 1.185287, 3.164869e-06, 191919.5, 0.0, 12.86659, 1.828514e-06], [52.0, 52.69421, 11.21244, 51.999, 52.67242, 0.04358434, 156.12, 1.342398, 51.99888, 52.0955, 52.34609, 51.99949, 52.46542, 52.67242, 2.286444, 1.075562, 2.081657e-06, 192439.7, 0.0, 11.76603, 2.789106e-06], [49.0, 49.61418, 9.645293, 49.001, 49.59518, 0.03799937, 156.0042, 1.162551, 48.99919, 49.13845, 49.32293, 49.00038, 49.4487, 49.59518, 2.049105, 0.9693383, 2.419945e-06, 192925.6, 0.0, 10.21014, 2.551699e-06], [46.0, 46.64398, 8.849838, 46.0014, 46.62327, 0.04141489, 155.8991, 1.162551, 45.99971, 46.20159, 46.31906, 45.99925, 46.54721, 46.62327, 1.829977, 0.8624549, 2.062263e-06, 193484.8, 0.0, 8.642792, 8.766135e-07], [43.0, 43.63805, 8.111564, 43.0, 43.61546, 0.04518427, 155.7963, 1.162551, 43.00087, 43.23263, 43.28277, 42.99939, 43.6105, 43.61546, 1.669476, 0.7863123, 2.202847e-06, 194031.9, 0.0, 8.304894, 2.187056e-06], [40.0, 40.60721, 7.850611, 39.9976, 40.58387, 0.04668618, 155.6928, 1.162551, 39.99903, 40.24392, 40.22946, 39.99922, 40.64502, 40.58387, 1.579687, 0.7417823, 1.934699e-06, 194511.3, 0.0, 7.823251, 1.052641e-06], [37.0, 37.55588, 7.570818, 37.0021, 37.53168, 0.04841156, 155.5887, 1.162551, 36.99997, 37.23081, 37.15568, 36.99985, 37.65521, 37.53168, 1.491856, 0.6986331, 1.616464e-06, 195029.6, 0.0, 7.701154, 1.426829e-06], [34.0, 34.39013, 7.129456, 34.002, 34.37085, 0.03855642, 155.4653, 1.006799, 34.00288, 34.19961, 34.07078, 33.99971, 34.53824, 34.37085, 1.389701, 0.6498903, 1.456064e-06, 195501.9, 0.0, 7.197325, 1.830936e-06], [31.0, 31.3295, 6.959681, 30.9971, 31.30975, 0.03949697, 155.3693, 1.006799, 31.00027, 31.15947, 30.98673, 30.99905, 31.52198, 31.30975, 1.305866, 0.6077944, 1.746532e-06, 195974.6, 0.0, 6.855044, 1.3535e-07], [28.0, 28.257, 6.444445, 28.0083, 28.23568, 0.04265477, 155.2754, 1.006799, 27.99751, 28.08427, 27.88122, 28.00025, 28.48138, 28.23568, 1.20443, 0.5603139, 1.207888e-06, 196438.7, 0.0, 6.465166, 2.29124e-06], [25.0, 25.1858, 5.908139, 25.0055, 25.16253, 0.04652672, 155.1906, 1.006799, 25.00147, 24.99086, 24.77406, 24.99832, 25.42586, 25.16253, 1.084087, 0.5032175, 9.614257e-07, 196931.6, 0.0, 5.92471, -5.51895e-08], [22.0, 22.16916, 5.305623, 21.9854, 22.14325, 0.05181037, 155.1142, 1.006799, 22.00671, 21.91764, 21.70696, 21.99982, 22.40575, 22.14325, 0.959603, 0.4446781, 7.916026e-07, 197380.4, 0.0, 5.277611, 2.768679e-07], [19.0, 19.30572, 4.637635, 18.9844, 19.27608, 0.05927295, 155.0499, 1.006799, 18.99661, 18.95241, 18.76765, 19.00061, 19.52011, 19.27608, 0.8426237, 0.390679, 5.587576e-07, 197860.4, 0.0, 4.670142, -7.621961e-08], [16.0, 16.50024, 3.972702, 16.0034, 16.46565, 0.06919378, 154.9962, 1.006799, 15.99681, 16.00464, 15.86607, 15.99389, 16.67341, 16.46565, 0.7071578, 0.3270905, 3.955843e-07, 198345.2, 0.0, 3.981336, -9.093087e-09], [13.0, 13.71888, 3.255681, 13.0265, 13.67666, 0.08443282, 154.9529, 1.006799, 12.99021, 12.98951, 12.9155, 12.99523, 13.83511, 13.67666, 0.5650661, 0.2606204, 4.899574e-08, 199058.5, 0.0, 3.267024, -3.089664e-07], [10.0, 11.02144, 2.634719, 9.9178, 10.96927, 0.1043323, 154.9244, 1.006799, 9.979209, 9.944225, 9.937939, 9.981572, 11.07989, 10.96927, 0.4191188, 0.1915213, 3.509129e-08, 199788.6, 0.0, 2.637912, 3.892924e-07], [7.0, 8.207977, 2.280254, 7.0263, 8.162771, 0.09041306, 154.877, 0.8719131, 6.996675, 6.899136, 6.944581, 6.995916, 8.207738, 8.162771, 0.272072, 0.1212537, 1.590448e-07, 200474.8, 0.0, 2.226699, -2.06841e-07], [4.0, 6.17061, 6.914511, 3.9852, 6.155702, 0.02981624, 154.8519, 0.8719131, 4.007358, 3.946248, 3.912001, 4.007225, 6.219766, 6.155702, 0.1566822, 0.06587024, 3.496313e-07, 201190.7, 0.0, 6.388795, -3.268214e-08], [2.0, 3.439481, -0.8426919, 2.2818, 3.470062, -0.06116255, 154.8119, 0.4359565, 2.275721, 2.314741, 2.136495, 2.275818, 3.587147, 3.470062, 0.06999886, 0.02771, -3.623877e-09, 201712.2, 0.0, -0.8426919, -3.623877e-09]]}])   [LabVIEW 2025]
uses:
  <vilib>/Analysis/6fits.llb/General Linear Fit Algorithm.ctl
  <vilib>/Analysis/NI_AALPro.lvlib
  <vilib>/Analysis/NI_AALBase.lvlib
panel:
  in  "sort with absolute\nx-value":bool
  in  "col. to be modified":u16=4
  out "processing":i32
  in  "algorithm":T1 items=["SVD", "Givens", "Givens2", "Householder", "LU Decomposition", "Cholesky", "SVD for Rank Deficient H"]
  in  "smooth factor":i32=121
  in  "iteration Number":i32=2
  in  "polynomial order":i32=2
  in  "filtering range":dbl
  in  "limit 2":dbl=0.0005 format="%.3e"
  in  "limit 1":dbl=0.0005 format="%.3e"
  out "note":string
  in  "menu":T2(ring)
  out "comparative":dbl
  in  "start processing":bool
  in  "sort column":u16=4
  # "(1) Data are sorted ascending or descending order.\n(2) Remove duplicate\n      i) Neighboring two data points are compared, if determined to be a duplicate, the second data point will be removed.\n      ii) Repeat i) unitl no duplicates found."
  # "Caution: All rows will be affected."
  # "(1) Select datasets to be processed"
  # "(Not the coulm of the plot but of the original dataset)"
  # "(2) Sort"
  # "i) Sort ?"
  # "ii) Ascending or descendingwhich order?"
  # "descending"
  # "(3)"
  # "(4) Start processing"
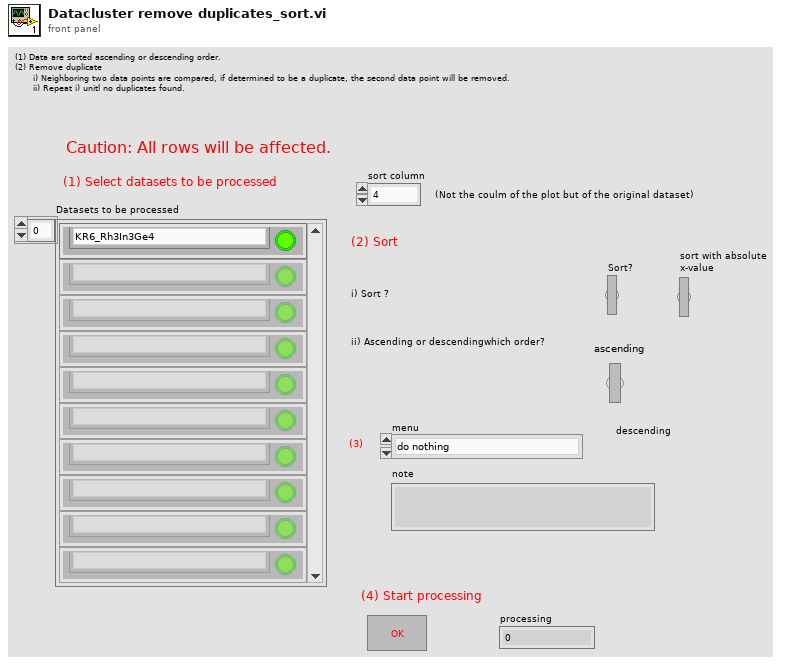
[diagram p1: front panel]
types:
  T1 = typedef "NI_AALPro.lvlib/General Linear Fit Algorithm.ctl" = u16
  T2 = enum16{"do nothing", "remove duplicates", "filtering out of the range", "remove glitches (poly. filter)", "remove glitches (boxcar. filter)", "smoothing only", "modify a column"}
  T3 = cluster{"String":string, "Boolean":bool, "begin":u32, "length":u32, "y weight":dbl}[]
  T4 = enum16{"do nothing", "remove duplicates", "filtering out of the range"}
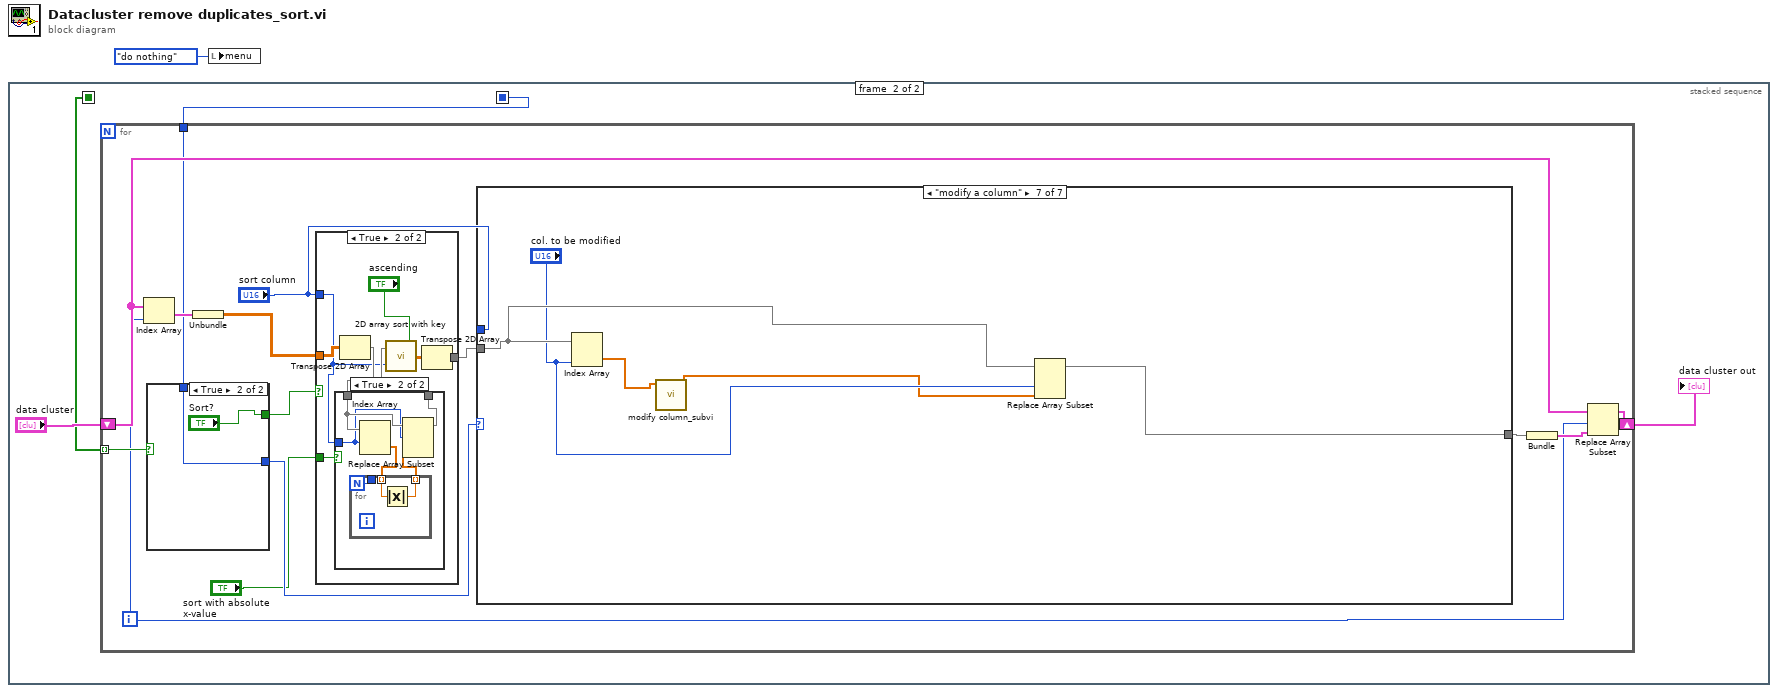
[diagram p0: block diagram]
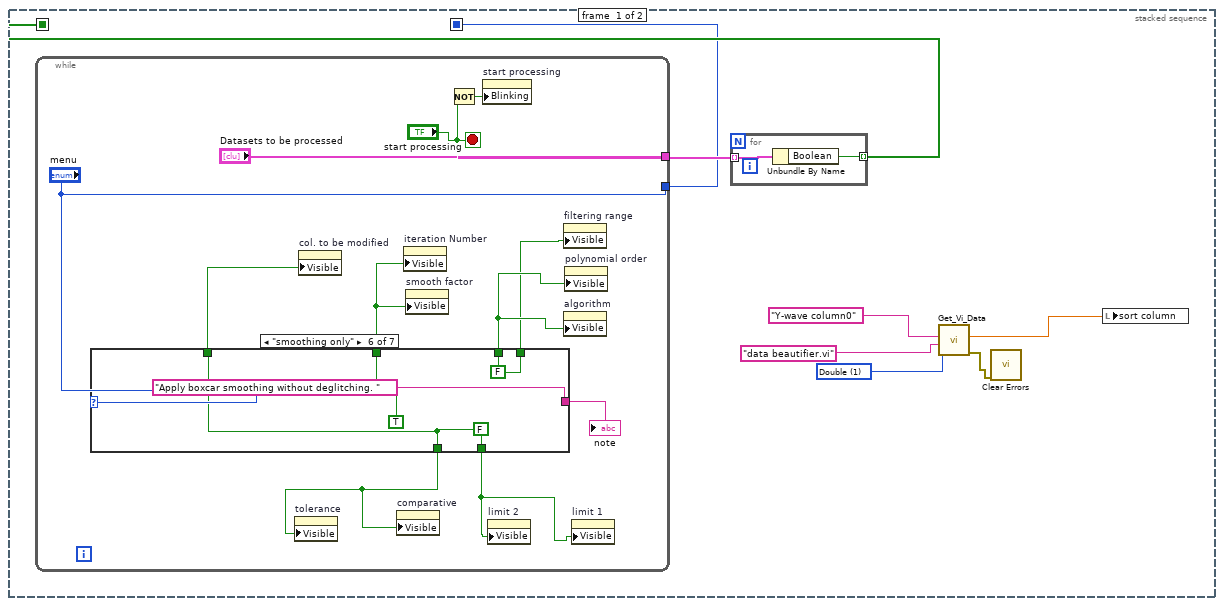
[diagram p2: hidden frame]
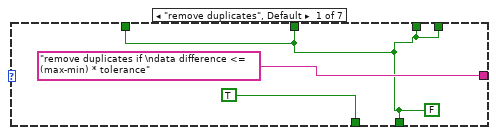
[diagram p3: hidden frame]
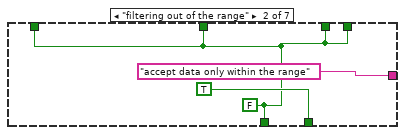
[diagram p4: hidden frame]
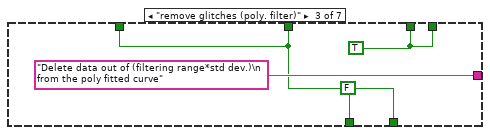
[diagram p5: hidden frame]
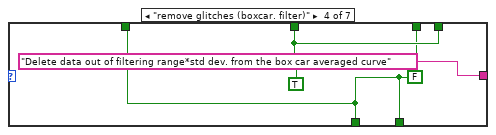
[diagram p6: hidden frame]
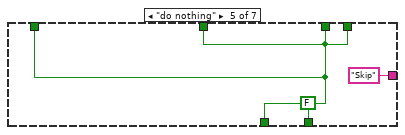
[diagram p7: hidden frame]
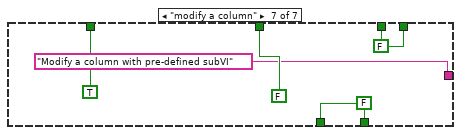
[diagram p8: hidden frame]
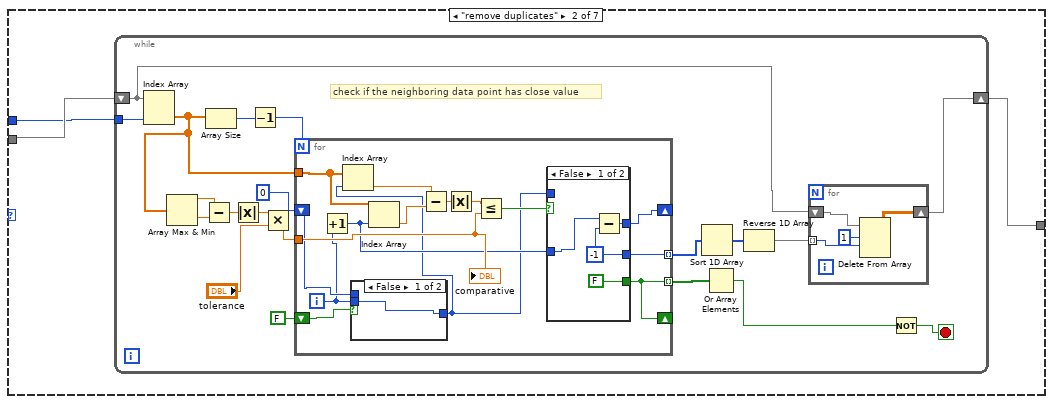
[diagram p10: hidden frame]
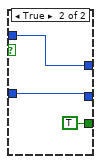
[diagram p12: hidden frame]
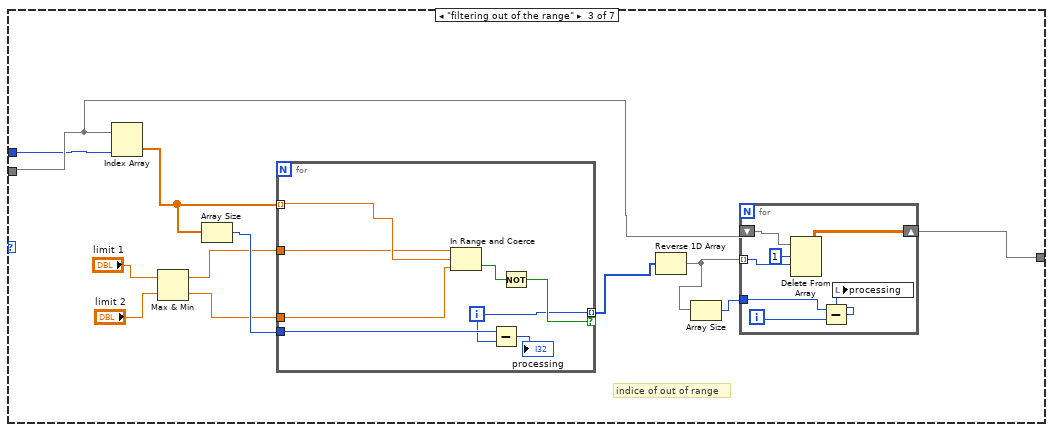
[diagram p13: hidden frame]
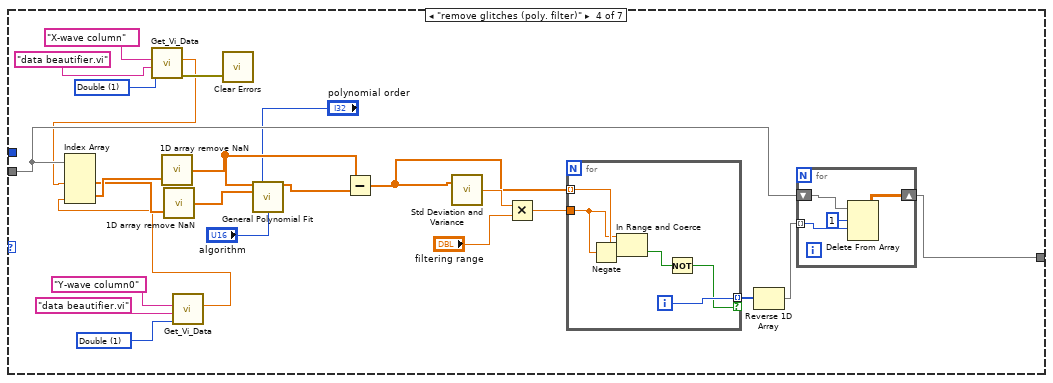
[diagram p14: hidden frame]
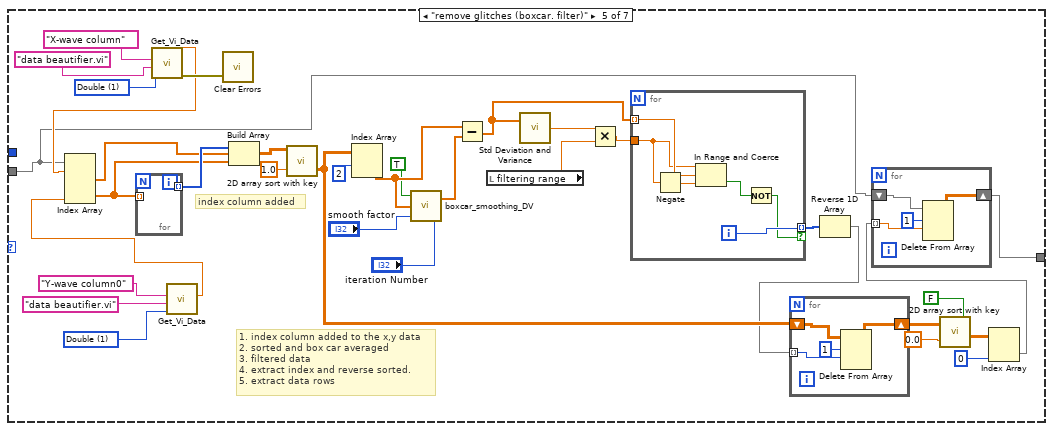
[diagram p15: hidden frame]
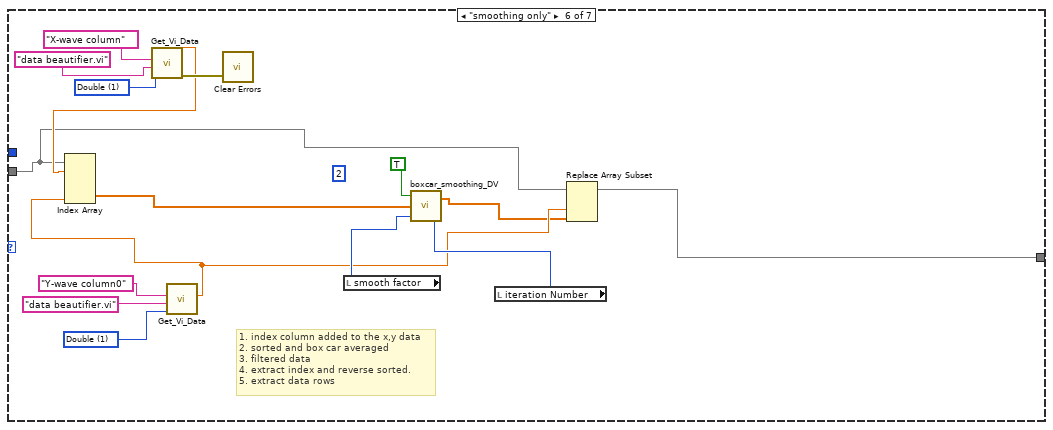
[diagram p16: hidden frame]
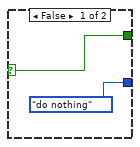
[diagram p17: hidden frame]
diagram:
  n1 = stacked-sequence {
    seq-local: [w8 _] -> [_ w47]
    seq-local: [w7 _] -> [_ w46]
    frame #0 {
      w4 = u16 1 items=["String", "Double", "Boolean", "Variant"] ("Data Type")
      n2 = while {
        tunnel: ["Datasets to be processed"] -> w9
        tunnel: ["menu"] -> w7
        stop <- "start processing" stop-if-true
        n3 = case shown="\"smoothing only\"" "menu" {
          tunnel: ["remove duplicates if \ndata difference <= (max-min) * tolerance" "accept data only within the range" "Delete data out of (filtering range*std dev.)\n from the poly fitted curve" "Delete data out of filtering range*std dev. from the box car averaged curve" "Skip" "Apply boxcar smoothing without deglitching. " "Modify a column with pre-defined subVI"] -> w18
          tunnel: [TRUE w26 w29 w32 w35 w37 w43] -> w17
          tunnel: [w23 TRUE w29 w32 w35 w37 w43] -> w16
          tunnel: [w23 w26 w30 w32 w35 w38 w42] -> w15
          tunnel: [w23 w26 w29 w33 w35 TRUE FALSE] -> w14
          tunnel: [w23 w26 w30 w33 w35 w38 w42] -> w13
          tunnel: [w23 w26 w29 w32 w35 w37 TRUE] -> w12
          frame "remove duplicates", Default {
            w23 = FALSE
          }
          frame "filtering out of the range" {
            w26 = FALSE
          }
          frame "remove glitches (poly. filter)" {
            w29 = FALSE
            w30 = TRUE
          }
          frame "remove glitches (boxcar. filter)" {
            w33 = TRUE
            w32 = FALSE
          }
          frame "do nothing" {
            w35 = FALSE
          }
          frame "smoothing only" {
            w37 = FALSE
            w38 = FALSE
          }
          frame "modify a column" {
            w43 = FALSE
            w42 = FALSE
          }
        }
        "note" <- w18
        n4 = property on="tolerance" class="DigNum (strict)"("Visible"=w17) -> ()  [unwired: 2 in, 2 out]
        n5 = property on="col. to be modified" class="DigNum (strict)"("Visible"=w12) -> ()  [unwired: 2 in, 2 out]
        n6 = property on="comparative" class="DigNum (strict)"("Visible"=w17) -> ()  [unwired: 2 in, 2 out]
        n7 = property on="iteration Number" class="DigNum (strict)"("Visible"=w14) -> ()  [unwired: 2 in, 2 out]
        n8 = property on="smooth factor" class="DigNum (strict)"("Visible"=w14) -> ()  [unwired: 2 in, 2 out]
        n9 = Not(x="start processing") -> (.not. x?=w21:bool)
        n10 = property on="start processing" class="Bool"("Blinking"=w21) -> ()  [unwired: 2 in, 2 out]
        n11 = property on="limit 2" class="DigNum (strict)"("Visible"=w16) -> ()  [unwired: 2 in, 2 out]
        n12 = property on="filtering range" class="DigNum (strict)"("Visible"=w13) -> ()  [unwired: 2 in, 2 out]
        n13 = property on="algorithm" class="Ring (strict)"("Visible"=w15) -> ()  [unwired: 2 in, 2 out]
        n14 = property on="polynomial order" class="DigNum (strict)"("Visible"=w15) -> ()  [unwired: 2 in, 2 out]
        n15 = property on="limit 1" class="DigNum (strict)"("Visible"=w16) -> ()  [unwired: 2 in, 2 out]
      }
      n16 = for {
        tunnel: w9 -> [w11] mode=indexing
        tunnel: [w10] -> w8 mode=indexing
        n17 = Unbundle By Name(w11) -> ("Boolean"=w10:bool)
      }
      n18 = call "Get_Vi_Data.vi"("Data Type"=w4, "VI name"="data beautifier.vi", "Control Name"="Y-wave column0") -> ("error out"=w2:errorcluster, "Data (Double)"=w3:dbl)  [unwired: 4 in, 3 out]
      n19 = call <vilib>:"Clear Errors.vi"("error in (no error)"=w2) -> ()  [unwired: 5 in, 2 out]
      n20 = local write "sort column"(w3) -> ()
    }
    frame #1 {
      n21 = for {
        shift-right: [w56] -> w48
        shift-left: "data cluster" -> [w59]
        tunnel: w47 -> [w55] mode=indexing
        tunnel: w46 -> [w53]
        i -> [w54]
        n22 = Index Array(array=w59, index=w54) -> (element=w62:cluster{"all rows":dbl[][]})
        n23 = case shown="True" w55 {
          selector: w55 -> [w249 _]
          tunnel: [w249 "Sort?"] -> w63
          tunnel: w53 -> [_ w250]
          tunnel: [T4."do nothing" ("menu") w250] -> w52
          frame False {
          }
          frame True {
          }
        }
        n24 = Unbundle(w62) -> ("all rows"=w61:dbl[][])
        n25 = case shown="True" w63 {
          tunnel: [w252 w257] -> w60
          tunnel: w61 -> [w252 w260]
          tunnel: "sort column" -> [_ w253]
          tunnel: "sort with absolute\nx-value" -> [_ w256]
          frame False {
          }
          frame True {
            n26 = Transpose 2D Array(2D array=w260) -> (transposed array=w254:dbl[][])
            n27 = case shown="True" w256 {
              tunnel: [w261 w262] -> w255
              tunnel: w254 -> [w261 w265]
              tunnel: w253 -> [_ w264]
              frame False {
              }
              frame True {
                n28 = Index Array(array=w265, index (row)=w264) -> (element=w266:dbl[])  [unwired: 1 in]
                n29 = for {
                  N -> [w269]
                  tunnel: [w269] -> _
                  tunnel: w266 -> [w268] mode=indexing
                  tunnel: [w267] -> w263 mode=indexing
                  n30 = Absolute Value(x=w268) -> (abs(x)=w267:dbl)
                }
                n31 = Replace Array Subset(array=w265, new element=w263, index (row)=w264) -> (w262:dbl[][])  [unwired: 1 in]
              }
            }
            n32 = call "2D array sort with key.vi"("ascending"="ascending", "key row"=w253, "input"=w255) -> ("output"=w259:dbl[][])
            n33 = Transpose 2D Array(2D array=w259) -> (transposed array=w257:dbl[][])
          }
        }
        n34 = case shown="\"modify a column\"" w52 {
          tunnel: [w64 w65 w125 w160 w208 w227 w246] -> w58
          tunnel: w60 -> [w64 w67 w127 w161 w178 w230 w247]
          tunnel: "sort column" -> [_ w66 w126 _ _ _ _]
          frame "do nothing", Default {
          }
          frame "remove duplicates" {
            n35 = while {
              tunnel: w66 -> [w81]
              shift-right: [w72] -> w65
              shift-left: w67 -> [w73]
              stop <- w82 stop-if-true
              # "check if the neighboring data point has close value"
              n36 = Index Array(array=w73, index (col)=w81) -> (element=w76:dbl[])  [unwired: 1 in]
              n37 = Array Max & Min(array=w76) -> (max value=w75:dbl, min value=w77:dbl)  [unwired: 2 out]
              n38 = Subtract(x=w75, y=w77) -> (x-y=w78:dbl)
              n39 = Array Size(array=w76) -> (size(s)=w71:i32)
              n40 = Absolute Value(x=w78) -> (abs(x)=w80:dbl)
              n41 = Decrement(x=w71) -> (x-1=w70:i32)
              n42 = Multiply(x=w80, y="tolerance") -> (x*y=w74:dbl)
              n43 = for {
                N: w70 -> [_]
                tunnel: w76 -> [w106]
                tunnel: w74 -> [w102]
                tunnel: [w97] -> w86 mode=indexing
                tunnel: [w98] -> w84 mode=indexing
                shift-right: [w96] -> _
                shift-left: 0 -> [w94]
                shift-right: [w98] -> _
                shift-left: FALSE -> [w95]
                i -> [w92]
                n44 = Increment(x=w92) -> (x+1=w100:i32)
                n45 = case shown="False" w95 {
                  tunnel: [w107 w108] -> w93
                  tunnel: w94 -> [_ w108]
                  tunnel: w92 -> [w107 _]
                  frame False {
                  }
                  frame True {
                  }
                }
                n46 = Index Array(array=w106, index=w93) -> (element=w104:dbl)
                n47 = Index Array(array=w106, index=w100) -> (element=w105:dbl)
                n48 = Subtract(x=w104, y=w105) -> (x-y=w103:dbl)
                n49 = Absolute Value(x=w103) -> (abs(x)=w99:dbl)
                n50 = Less Or Equal?(x=w99, y=w102) -> (x <= y?=w101:bool)
                n51 = case shown="False" w101 {
                  tunnel: w100 -> [w110 w115]
                  tunnel: [w111 w115] -> w97
                  tunnel: [FALSE TRUE] -> w98
                  tunnel: [w109 w113] -> w96
                  tunnel: w93 -> [_ w113]
                  frame False {
                    w111 = -1
                    n52 = Subtract(x=w110, y=w111) -> (x-y=w109:i32)
                  }
                  frame True {
                  }
                }
                "comparative" <- w102
              }
              n53 = Sort 1D Array(array=w86) -> (sorted array=w87:i32[])
              n54 = Or Array Elements(Boolean array=w84) -> (logical OR=w83:bool)
              n55 = Reverse 1D Array(array=w87) -> (reversed array=w85:i32[])
              n56 = for {
                tunnel: w85 -> [w90] mode=indexing
                shift-right: [w88] -> w72
                shift-left: w73 -> [w89]
                n57 = Delete From Array(array=w89, length=1, index (row)=w90) -> (array with subset deleted=w88:dbl[][])  [unwired: 1 in, 1 out]
              }
              n58 = Not(x=w83) -> (.not. x?=w82:bool)
            }
          }
          frame "filtering out of the range" {
            # "indice of out of range"
            n59 = Index Array(array=w127, index (col)=w126) -> (element=w123:dbl[])  [unwired: 1 in]
            n60 = Max & Min(x="limit 1", y="limit 2") -> (max(x,y)=w118:dbl, min(x,y)=w116:dbl)
            n61 = Array Size(array=w123) -> (size(s)=w122:i32)
            n62 = for {
              tunnel: w123 -> [w140] mode=indexing
              tunnel: [w138] -> w124 mode=indexing if=w141
              tunnel: w122 -> [w139]
              tunnel: w118 -> [w136]
              tunnel: w116 -> [w135]
              i -> [w138]
              n63 = In Range and Coerce(upper limit=w136, x=w140, lower limit=w135) -> (In Range?=w142:bool)  [unwired: 1 out]
              n64 = Subtract(x=w139, y=w138) -> (x-y=→"processing":i32)
              n65 = Not(x=w142) -> (.not. x?=w141:bool)
            }
            n66 = Reverse 1D Array(array=w124) -> (reversed array=w121:i32[])
            n67 = Array Size(array=w121) -> (size(s)=w120:i32)
            n68 = for {
              tunnel: w121 -> [w133] mode=indexing
              shift-right: [w131] -> w125
              shift-left: w127 -> [w132]
              tunnel: w120 -> [w130]
              i -> [w129]
              n69 = Delete From Array(array=w132, length=1, index (row)=w133) -> (array with subset deleted=w131:dbl[][])  [unwired: 1 in, 1 out]
              n70 = Subtract(x=w130, y=w129) -> (x-y=w128:i32)
              n71 = local write "processing"(w128) -> ()
            }
          }
          frame "remove glitches (poly. filter)" {
            w145 = u16 1 items=["String", "Double", "Boolean", "Variant"] ("Data Type")
            w157 = u16 1 items=["String", "Double", "Boolean", "Variant"] ("Data Type")
            n72 = call "Get_Vi_Data.vi"("Data Type"=w157, "VI name"="data beautifier.vi", "Control Name"="X-wave column") -> ("error out"=w156:errorcluster, "Data (Double)"=w154:dbl)  [unwired: 4 in, 3 out]
            n73 = call "Get_Vi_Data.vi"("Data Type"=w145, "VI name"="data beautifier.vi", "Control Name"="Y-wave column0") -> ("Data (Double)"=w143:dbl)  [unwired: 4 in, 4 out]
            n74 = Index Array(array=w161, index (col) #1=w154, index (col) #2=w143) -> (element #1=w151:dbl[], element #2=w153:dbl[])  [unwired: 2 in]
            n75 = call "1D array remove NaN.vi"("Array input"=w153) -> ("cleaned array"=w152:dbl[])  [unwired: 1 in]
            n76 = call "1D array remove NaN.vi"("Array input"=w151) -> ("cleaned array"=w148:dbl[])  [unwired: 1 in]
            n77 = call <vilib>:"Clear Errors.vi"("error in (no error)"=w156) -> ()  [unwired: 5 in, 2 out]
            n78 = call <vilib>:"General Polynomial Fit.vi"("Y"=w152, "polynomial order"="polynomial order", "X"=w148, "algorithm"="algorithm") -> ("Best Polynomial Fit"=w149:dbl[])  [unwired: 8 in, 3 out]
            n79 = Subtract(x=w152, y=w149) -> (x-y=w155:dbl[])
            n80 = call <vilib>:"Std Deviation and Variance.vi"("X"=w155) -> ("standard deviation"=w166:dbl)  [unwired: 1 in, 2 out]
            n81 = Multiply(x=w166, y="filtering range") -> (x*y=w164:dbl)
            n82 = for {
              tunnel: w155 -> [w173] mode=indexing
              tunnel: [w176] -> w162 mode=indexing if=w174
              tunnel: w164 -> [w172]
              i -> [w176]
              n83 = Negate(x=w172) -> (-x=w171:dbl)
              n84 = In Range and Coerce(upper limit=w172, x=w173, lower limit=w171) -> (In Range?=w175:bool)  [unwired: 1 out]
              n85 = Not(x=w175) -> (.not. x?=w174:bool)
            }
            n86 = Reverse 1D Array(array=w162) -> (reversed array=w163:i32[])
            n87 = for {
              tunnel: w163 -> [w169] mode=indexing
              shift-right: [w167] -> w160
              shift-left: w161 -> [w168]
              n88 = Delete From Array(array=w168, length=1, index (row)=w169) -> (array with subset deleted=w167:dbl[][])  [unwired: 1 in, 1 out]
            }
          }
          frame "remove glitches (boxcar. filter)" {
            w188 = u16 1 items=["String", "Double", "Boolean", "Variant"] ("Data Type")
            w205 = u16 1 items=["String", "Double", "Boolean", "Variant"] ("Data Type")
            # "1. index column added to the x,y data\n2. sorted and box car averaged\n3. filtered data\n4. extract index and reverse sorted.\n5. extract data rows"
            # "index column added"
            n89 = call "Get_Vi_Data.vi"("Data Type"=w205, "VI name"="data beautifier.vi", "Control Name"="X-wave column") -> ("error out"=w204:errorcluster, "Data (Double)"=w197:dbl)  [unwired: 4 in, 3 out]
            n90 = call "Get_Vi_Data.vi"("Data Type"=w188, "VI name"="data beautifier.vi", "Control Name"="Y-wave column0") -> ("Data (Double)"=w186:dbl)  [unwired: 4 in, 4 out]
            n91 = Index Array(array=w178, index (col) #1=w197, index (col) #2=w186) -> (element #1=w195:dbl[], element #2=w196:dbl[])  [unwired: 2 in]
            n92 = for {
              tunnel: w196 -> [_] mode=indexing
              tunnel: [w216] -> w203 mode=indexing
              i -> [w216]
            }
            n93 = call <vilib>:"Clear Errors.vi"("error in (no error)"=w204) -> ()  [unwired: 5 in, 2 out]
            n94 = Build Array(w203, w195, w196) -> (w202:dbl[][])
            n95 = call "2D array sort with key.vi"("key row"=1.0, "input"=w202) -> ("output"=w185:dbl[][])  [unwired: 1 in]
            n96 = Index Array(array=w185, index (row)=2 ("disabled index (col)")) -> (element=w193:dbl[])  [unwired: 1 in]
            n97 = call "boxcar_smoothing_DV.vi"("iteration Number"="iteration Number", "smooth factor"="smooth factor", "raw data"=w193, "NaN filter"=TRUE) -> ("smoothed"=w194:dbl[])
            n98 = Subtract(x=w193, y=w194) -> (x-y=w192:dbl[])
            n99 = local read "filtering range"() -> (w191:dbl)
            n100 = call <vilib>:"Std Deviation and Variance.vi"("X"=w192) -> ("standard deviation"=w211:dbl)  [unwired: 1 in, 2 out]
            n101 = Multiply(x=w211, y=w191) -> (x*y=w210:dbl)
            n102 = for {
              tunnel: w192 -> [w223] mode=indexing
              tunnel: [w226] -> w209 mode=indexing if=w224
              tunnel: w210 -> [w222]
              i -> [w226]
              n103 = Negate(x=w222) -> (-x=w221:dbl)
              n104 = In Range and Coerce(upper limit=w222, x=w223, lower limit=w221) -> (In Range?=w225:bool)  [unwired: 1 out]
              n105 = Not(x=w225) -> (.not. x?=w224:bool)
            }
            n106 = Reverse 1D Array(array=w209) -> (reversed array=w184:i32[])
            n107 = for {
              tunnel: w184 -> [w214] mode=indexing
              shift-right: [w212] -> w183
              shift-left: w185 -> [w213]
              n108 = Delete From Array(array=w213, length=1, index (row)=w214) -> (array with subset deleted=w212:dbl[][])  [unwired: 1 in, 1 out]
            }
            n109 = call "2D array sort with key.vi"("ascending"=FALSE, "key row"=0.0, "input"=w183) -> ("output"=w181:dbl[][])
            n110 = Index Array(array=w181, index (row)=0) -> (element=w179:dbl[])  [unwired: 1 in]
            n111 = for {
              tunnel: w179 -> [w219] mode=indexing
              shift-right: [w217] -> w208
              shift-left: w178 -> [w218]
              n112 = Delete From Array(array=w218, length=1, index (row)=w219) -> (array with subset deleted=w217:dbl[][])  [unwired: 1 in, 1 out]
            }
          }
          frame "smoothing only" {
            w235 = u16 1 items=["String", "Double", "Boolean", "Variant"] ("Data Type")
            (unwired) 2 ("disabled index (col)")
            w240 = u16 1 items=["String", "Double", "Boolean", "Variant"] ("Data Type")
            # "1. index column added to the x,y data\n2. sorted and box car averaged\n3. filtered data\n4. extract index and reverse sorted.\n5. extract data rows"
            n113 = call "Get_Vi_Data.vi"("Data Type"=w240, "VI name"="data beautifier.vi", "Control Name"="X-wave column") -> ("error out"=w239:errorcluster, "Data (Double)"=w238:dbl)  [unwired: 4 in, 3 out]
            n114 = call "Get_Vi_Data.vi"("Data Type"=w235, "VI name"="data beautifier.vi", "Control Name"="Y-wave column0") -> ("Data (Double)"=w229:dbl)  [unwired: 4 in, 4 out]
            n115 = Index Array(array=w230, index (col) #1=w238, index (col) #2=w229) -> (element #2=w231:dbl[])  [unwired: 2 in, 1 out]
            n116 = call <vilib>:"Clear Errors.vi"("error in (no error)"=w239) -> ()  [unwired: 5 in, 2 out]
            n117 = local read "smooth factor"() -> (w233:i32)
            n118 = local read "iteration Number"() -> (w232:i32)
            n119 = call "boxcar_smoothing_DV.vi"("iteration Number"=w232, "smooth factor"=w233, "raw data"=w231, "NaN filter"=TRUE) -> ("smoothed"=w228:dbl[])
            n120 = Replace Array Subset(array=w230, new element=w228, index (col)=w229) -> (w227:dbl[][])  [unwired: 1 in]
          }
          frame "modify a column" {
            n121 = Index Array(array=w247, index (col)="col. to be modified") -> (element=w245:dbl[])  [unwired: 1 in]
            n122 = call "modify column_subvi.vi"("array in"=w245) -> ("array out"=w243:dbl[])  [unwired: 10 in]
            n123 = Replace Array Subset(array=w247, new element=w243, index (col)="col. to be modified") -> (w246:dbl[][])  [unwired: 1 in]
          }
        }
        n124 = Bundle("all rows"=w58) -> (w57:cluster{"all rows":dbl[][]})  [unwired: 1 in]
        n125 = Replace Array Subset(array=w59, new element=w57, index=w54) -> (w56:cluster{"all rows":dbl[][]}[])
      }
      "data cluster out" <- w48
    }
  }
  n126 = local write "menu"(T2."do nothing" ("menu")) -> ()
